vi "Array-Dimensions (3D).vi"(7 "3D Array":dbl[][][](array[numeric])) -> (4 "# pages":i32, 8 "# rows":i32, 15 "# columns":i32)   [LabVIEW 2020]
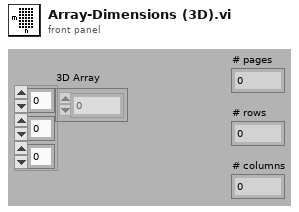
[diagram p1: front panel]
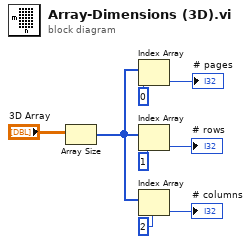
[diagram p0: block diagram]
diagram:
  n1 = Array Size(array="3D Array") -> (size(s)=w4:i32[])
  n2 = Index Array(array=w4, index=0) -> (element=→"# pages":i32)
  n3 = Index Array(array=w4, index=1) -> (element=→"# rows":i32)
  n4 = Index Array(array=w4, index=2) -> (element=→"# columns":i32)
